vi "4.2 Surface Area and Volume of a Sphere-Prob2.vi"() -> ()   [LabVIEW 2025]
panel:
  out "Boolean":bool
  out "Random Number 2":dbl(knob) scale=0.0..1.0
  out "Random Number 1":dbl(knob) scale=0.0..1.0
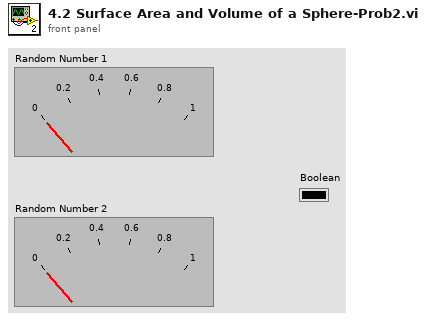
[diagram p1: front panel]
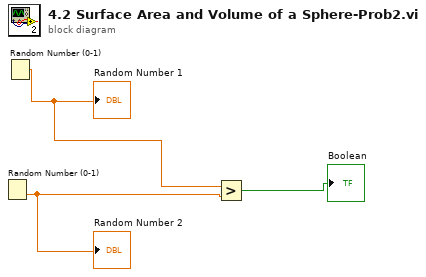
[diagram p0: block diagram]
diagram:
  n1 = Random Number (0-1)() -> (number: 0 to 1=w2:dbl)
  "Random Number 2" <- w2
  n2 = Random Number (0-1)() -> (number: 0 to 1=w1:dbl)
  "Random Number 1" <- w1
  n3 = Greater?(x=w1, y=w2) -> (0:→"Boolean":bool)
